vi "DeCoF wait for prompt ASRL.vi"(6 "error in (no error)":errorcluster, 7 "time out (ms)":i32=1000, 9 "VISA resource name":refnum<visa-resource-name>) -> (0 "error out":errorcluster, 1 "timed out?":bool, 2 "answer string":string, 3 "VISA resource name out":refnum<visa-resource-name>, 4 "complete answer":string)   [LabVIEW 2013]
doc: "This VI collects the input from the serial connection until the prompt string is found or the timeout expires.\nThe answer string contains the complete collected string minus the prompt, if found."
uses:
  <vilib>/Instr/_visa.llb/Select Event Type.ctl
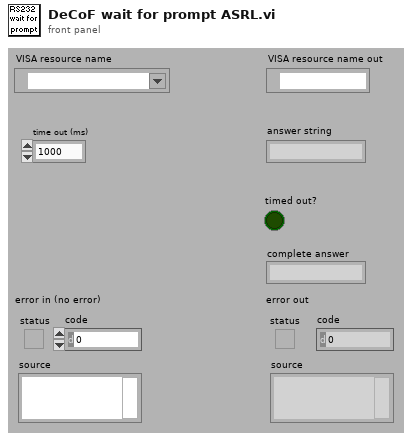
[diagram p1: front panel]
types:
  T1 = typedef "Select Event Type.ctl" = u32
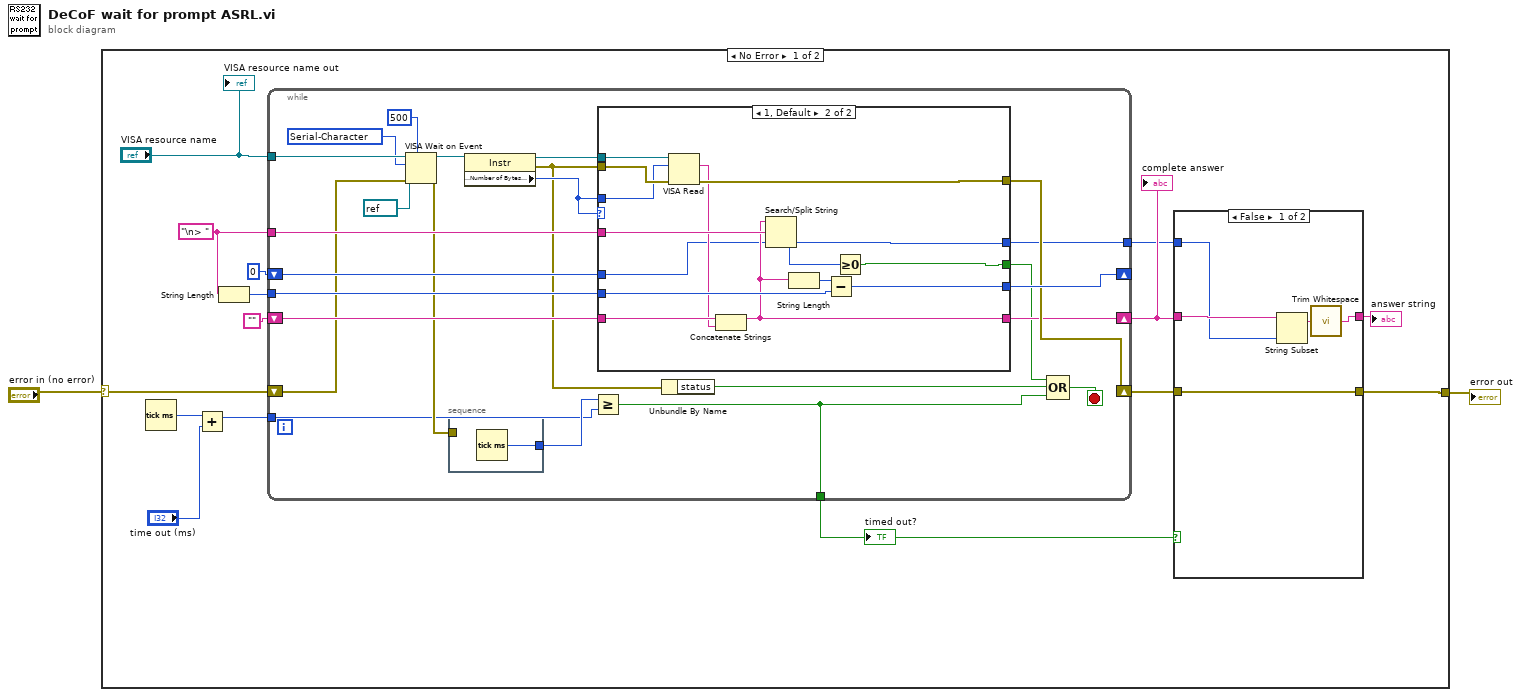
[diagram p0: block diagram]
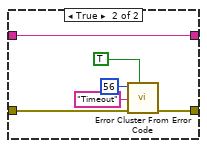
[diagram p2: hidden frame]
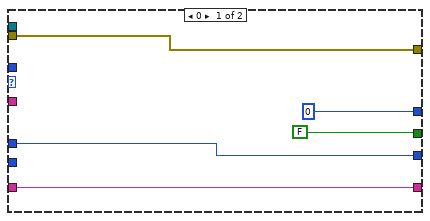
[diagram p3: hidden frame]
diagram:
  n1 = case shown="No Error" "error in (no error)" {
    selector: "error in (no error)" -> [w16 w73]
    tunnel: [w11 w73] -> w1
    frame No Error {
      w15 = "\n> " ("prompt")
      n2 = Tick Count (ms)() -> (millisecond timer value=w7:u32)
      n3 = Add(x=w7, y="time out (ms)") -> (x+y=w5:u32)
      n4 = String Length(string=w15) -> (length=w8:i32)
      n5 = while {
        shift-right: [w46] -> w12
        shift-left: w16 -> [w37]
        tunnel: "VISA resource name" -> [w36]
        tunnel: w5 -> [w31]
        shift-right: [w49] -> _
        shift-left: 0 -> [w51]
        tunnel: w15 -> [w50]
        tunnel: w8 -> [w48]
        shift-right: [w44] -> w13
        shift-left: "" -> [w45]
        tunnel: [w39] -> w9
        tunnel: [w30] -> w4
        stop <- w47 stop-if-true
        w29 = T1 1073684533 items=["ServiceRequest"=1073684491, "Trigger"=3221168138, "Clear"=1073684493, "VXI-Signal"=1073684512, "VXI/VME-Interrupt"=3221168161, "VXI/VME-Sysfail"=1073684509, "VXI/VME-Sysreset"=1073684510, "GPIB-CIC"=1073684498, "GPIB-Talk"=1073684499, "GPIB-Listen"=1073684500, "PXI-Interrupt"=1073684514, "Serial-Break"=1073684515, "Serial-TermChar"=1073684516, "Serial-CTS"=1073684521, "Serial-DSR"=1073684522, "Serial-DCD"=1073684524, "Serial-RI"=1073684526, "Serial-Character"=1073684533, "USB-Interrupt"=1073684535, "AllEnabled"=1073709055] ("Event Type")
        n6 = VISA Wait on Event(7:u32 500 ("timeout (0)"), 8:w37, 9:refnum<visa-resource-name> refnum ("event resource class"), 10:w29, 11:w36) -> (0:w34:errorcluster, 3:w38:refnum<visa-resource-name>)  [unwired: 2 out]
        n7 = stacked-sequence {
          tunnel: w34 -> [_]
          tunnel: [w53] -> w35
          frame #0 {
            n8 = Tick Count (ms)() -> (millisecond timer value=w53:u32)
          }
        }
        n9 = property class="Instr"(reference=w38) -> (reference out=w52:refnum<visa-resource-name>, error out=w33:errorcluster, "Serial Settings:Number of Bytes at Serial Port"=w41:u32)  [unwired: 1 in]
        n10 = Greater Or Equal?(x=w35, y=w31) -> (x >= y?=w30:bool)
        n11 = case shown="1, Default" w41 {
          tunnel: w52 -> [_ w72]
          tunnel: w33 -> [w58 w71]
          tunnel: w41 -> [_ w70]
          tunnel: w51 -> [w57 w60]
          tunnel: w50 -> [_ w69]
          tunnel: [w57 w63] -> w49
          tunnel: w48 -> [_ w68]
          tunnel: [w58 w67] -> w46
          tunnel: w45 -> [w56 w66]
          tunnel: [w56 w61] -> w44
          tunnel: [FALSE w62] -> w40
          tunnel: [0 ("offset of match") w59] -> w39
          frame 0 {
          }
          frame 1, Default {
            n12 = VISA Read(VISA resource name=w72, byte count=w70, error in (no error)=w71) -> (read buffer=w65:string, error out=w67:errorcluster)  [unwired: 2 out]
            n13 = Concatenate Strings(w66, w65) -> (w61:string)
            n14 = Search/Split String(string=w61, search string/char (-)=w69, offset (0)=w60) -> (offset of match=w59:i32)  [unwired: 2 out]
            n15 = String Length(string=w61) -> (length=w64:i32)
            n16 = Subtract(x=w64, y=w68) -> (x-y=w63:i32)
            n17 = Greater Or Equal To 0?(x=w59) -> (x >= 0?=w62:bool)
          }
        }
        n18 = Unbundle By Name(w33) -> ("status"=w32:bool)
        n19 = Compound Arithmetic op=OR(w40, w32, w30) -> (w47:bool)
      }
      "timed out?" <- w4
      "complete answer" <- w13
      n20 = case shown="False" w4 {
        tunnel: w13 -> [w22 w28]
        tunnel: [w20 w28] -> w10
        tunnel: [w19 w26] -> w11
        tunnel: w12 -> [w19 w27]
        tunnel: w9 -> [w18 _]
        frame False {
          n21 = String Subset(string=w22, length (rest)=w18) -> (substring=w21:string)  [unwired: 1 in]
          n22 = call <vilib>:"Trim Whitespace.vi"("string"=w21) -> ("trimmed string"=w20:string)  [unwired: 1 in]
        }
        frame True {
          n23 = call <vilib>:"Error Cluster From Error Code.vi"("show call chain? (False)"=TRUE, "error in (no error)"=w27, "error message (\"\")"="Timeout" ("error message (\"\")"), "error code (0)"=56) -> ("error out"=w26:errorcluster)  [unwired: 5 in]
        }
      }
      "answer string" <- w10
      "VISA resource name out" <- "VISA resource name"
    }
    frame Error {
    }
  }
  "error out" <- w1
